vi "Remove Contact.vi"(8 "error in (no error)":errorcluster) -> (0 "error out":errorcluster)   [LabVIEW 2014, in "Map Data.lvlib"]
doc: "Removes a contact from the address book data store."
uses:
  Map Data.lvlib
  MapCommand.ctl
  MapDatas.ctl
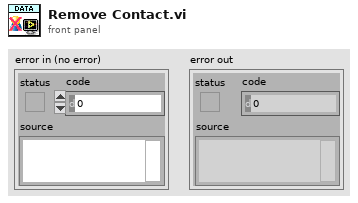
[diagram p1: front panel]
types:
  T1 = typedef "Map Data.lvlib/MapDatas.ctl" = cluster{"X":dbl, "Y":dbl, "Z":dbl, "heading":dbl, "X2":dbl, "Y2":dbl, "Z2":dbl}
  T2 = typedef "Map Data.lvlib/MapCommand.ctl" = enum16{"Load", "Update Cursor", "Save", "Get All Data", "Get Single Data", "Set Single Data", "Delete All", "Remove Single Data", "Set Favorite Status", "Is Data Modified", "Import Data"}
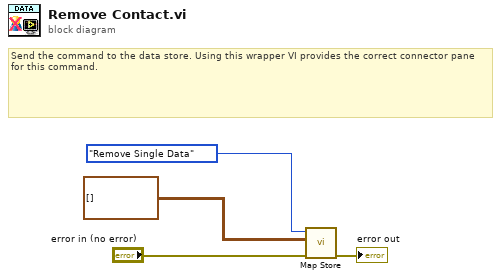
[diagram p0: block diagram]
diagram:
  # "Send the command to the data store. Using this wrapper VI provides the correct connector pane for this command."
  n1 = call "Map Store.vi"("error in (no error)"="error in (no error)", "All Lines"=T1[][] [], "Command"=MapCommand."Remove Single Data") -> ("error out"=→"error out":errorcluster)  [unwired: 5 in, 3 out]
